vi "LoadCalcFunc.vi"(4 "InstrPar":T1, 6 "Operation Name":string, 8 "ErrorIn(No Error)":errorcluster caption="entrée d'erreur (pas d'erreur)", 9 "DataQNames":string[](array[string]), 10 "Calc_Func":T2, 11 "Experiment.lvclass":refnum<class "Experiment.lvclass">) -> (0 "sortie d'erreur":errorcluster, 1 "LoadedTools":refnum<class "BaseDevice.lvclass">[](array[class]), 2 "ToolIndex":i32, 3 "Experiment.lvclass Out":refnum<class "Experiment.lvclass">)   [LabVIEW 2019, in "Experiment.lvclass"]
uses:
  Experiment.lvclass
  Calculations Class/DefaultDev_Func.ctl
  DevicesClass/BaseDevice/BaseDevice.lvclass
  Experiment.lvclass/Experiment.ctl
  Calculations Class/Calculations.lvclass
  C:/Programmes Labview/LabScanV1A/DevicesClass/BaseDevice/BaseDevice.lvclass
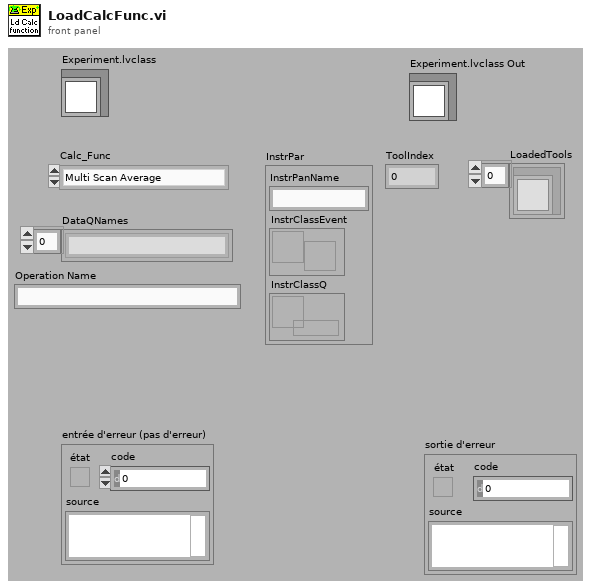
[diagram p1: front panel]
types:
  T1 = cluster{"InstrPanName":string, "InstrClassEvent":refnum<user-event>, "InstrClassQ":refnum<queue>}
  T2 = typedef "Calculations.lvclass/DefaultDev_Func.ctl" = enum16{"Multi Scan Average", "Running Average", "Summ"}
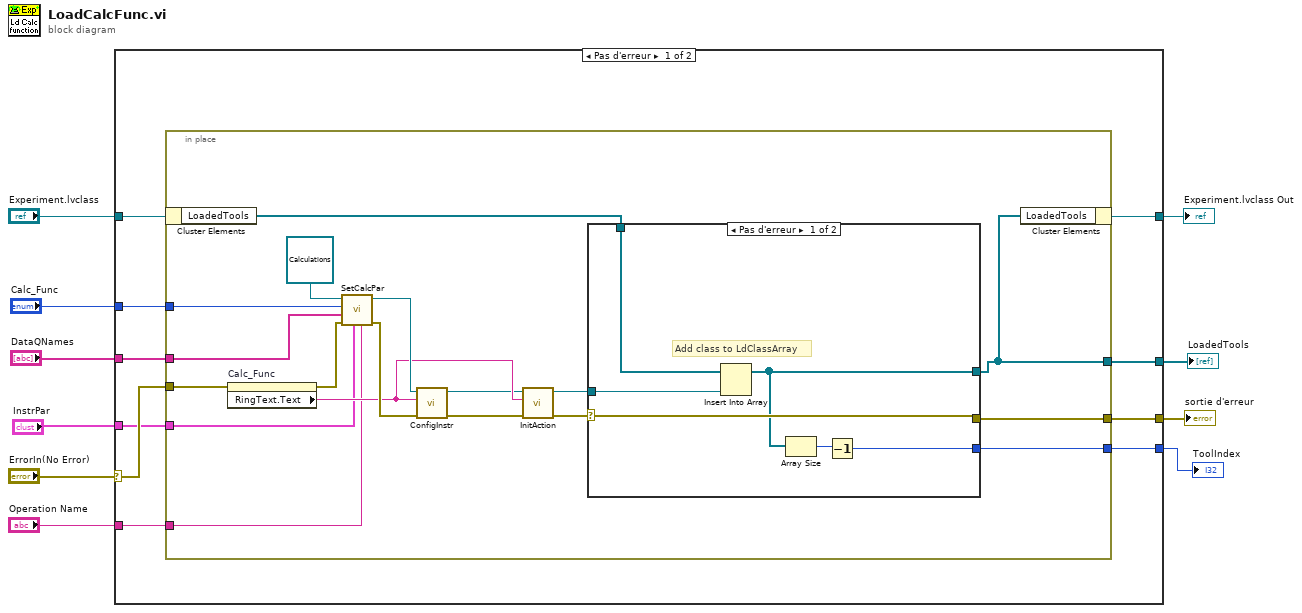
[diagram p0: block diagram]
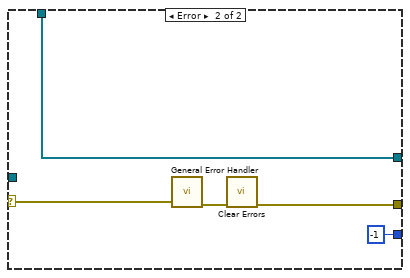
[diagram p2: hidden frame]
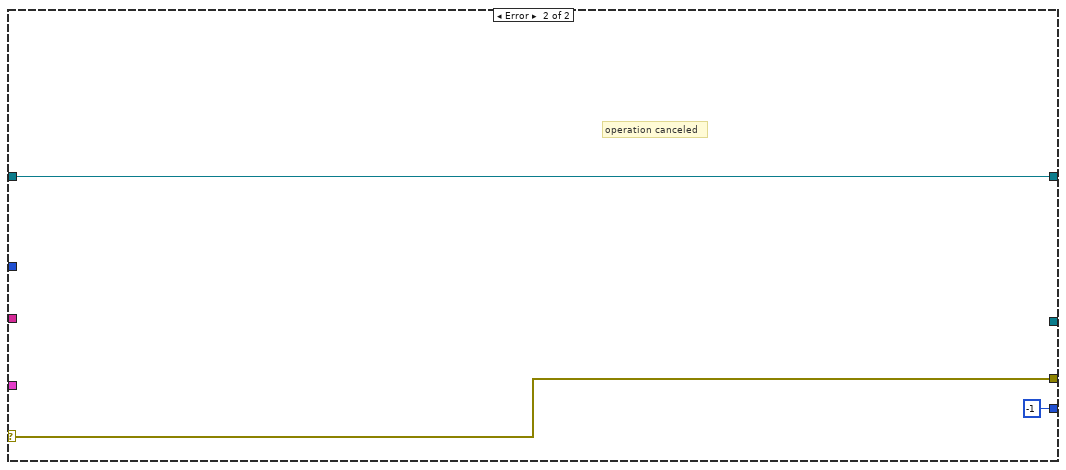
[diagram p3: hidden frame]
diagram:
  n1 = case shown="Pas d'erreur" "ErrorIn(No Error)" {
    selector: "ErrorIn(No Error)" -> [w19 w52]
    tunnel: [w17 w52] -> w9
    tunnel: "Experiment.lvclass" -> [w18 w51]
    tunnel: [w16 w51] -> w7
    tunnel: "Calc_Func" -> [w20 _]
    tunnel: "DataQNames" -> [w15 _]
    tunnel: "InstrPar" -> [w14 _]
    tunnel: [w13 -1] -> w4
    tunnel: [w12 _] -> w3
    tunnel: "Operation Name" -> [w11 _]
    frame No Error {
      n2 = in-place {
        in-place-border: w20 -> [w36]
        in-place-border: w19 -> [w34]
        in-place-border: [w29] -> w17
        in-place-border: w15 -> [w28]
        in-place-border: w14 -> [w26]
        in-place-border: [w25] -> w13
        in-place-border: [w24] -> w12
        in-place-border: w11 -> [w21]
        n3 = in-place-cluster #1(w18) -> ("LoadedTools"=w31:refnum<class "BaseDevice.lvclass">[])
        n4 = property on="Calc_Func" class="Énum (strict)"(error in=w34) -> (error out=w33:errorcluster, "RingText.Text"=w27:string)  [unwired: 1 in, 1 out]
        n5 = call "SetCalcPar.vi"("Operation Name"=w21, "InstrPar"=w26, "error in (no error)"=w33, "DataQNames"=w28, "Calc_Func"=w36, "GenData In"=refnum<class "Calculations.lvclass"> refnum ("Calculations.lvclass")) -> ("error out"=w35:errorcluster, "GenData Out"=w37:refnum<class "Calculations.lvclass">)  [unwired: 4 in]
        n6 = call-dynamic "ConfigInstr.vi"("error in (no error)"=w35, "Function"=w27, "GenData In"=w37) -> ("error out"=w23:errorcluster, "GenData Out"=w22:refnum<class "Calculations.lvclass">)  [unwired: 7 in]
        n7 = call-dynamic "InitAction.vi"("error in (no error)"=w23, "Function"=w27, "GenData In"=w22) -> ("error out"=w32:errorcluster, "GenData Out"=w30:refnum<class "Calculations.lvclass">)  [unwired: 7 in]
        n8 = case shown="Pas d'erreur" w32 {
          selector: w32 -> [w43 w48]
          tunnel: w31 -> [w44 w49]
          tunnel: w30 -> [w42 _]
          tunnel: [w41 w49] -> w24
          tunnel: [w43 w46] -> w29
          tunnel: [w39 -1] -> w25
          frame No Error {
            # "Add class to LdClassArray"
            n9 = Insert Into Array(array=w44, new element=w42) -> (w41:refnum<class "BaseDevice.lvclass">[])  [unwired: 1 in]
            n10 = Array Size(array=w41) -> (size(s)=w40:i32)
            n11 = Decrement(x=w40) -> (x-1=w39:i32)
          }
          frame Error {
            n12 = call <vilib>:"General Error Handler.vi"("error in (no error)"=w48) -> ("error out"=w47:errorcluster)  [unwired: 10 in, 4 out]
            n13 = call <vilib>:"Clear Errors.vi"("error in (no error)"=w47) -> ("error out"=w46:errorcluster)  [unwired: 5 in, 1 out]
          }
        }
        n14 = in-place-cluster #1("LoadedTools"=w24) -> (w16:refnum<class "Experiment.lvclass">)
      }
    }
    frame Error {
      # "operation canceled"
    }
  }
  "sortie d'erreur" <- w9
  "Experiment.lvclass Out" <- w7
  "ToolIndex" <- w4
  "LoadedTools" <- w3
